vi "Limelight Aim & Range.vi"() -> (2 "Right command":dbl, 3 "left command":dbl)   [LabVIEW 2019]
uses:
  Framework/Robot Global Data.vi
panel:
  out "tv - valid target":dbl=1.0
  out "ty - offsetAngle V":dbl=-1.5031967163085938
  out "tx - offsetAngle H":dbl=0.16126251220703125
  out "distance adjust":dbl
  out "steering adjust":dbl
  out "heading error":dbl
  out "distance error":dbl
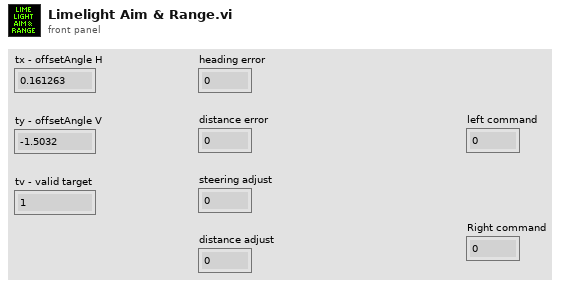
[diagram p1: front panel]
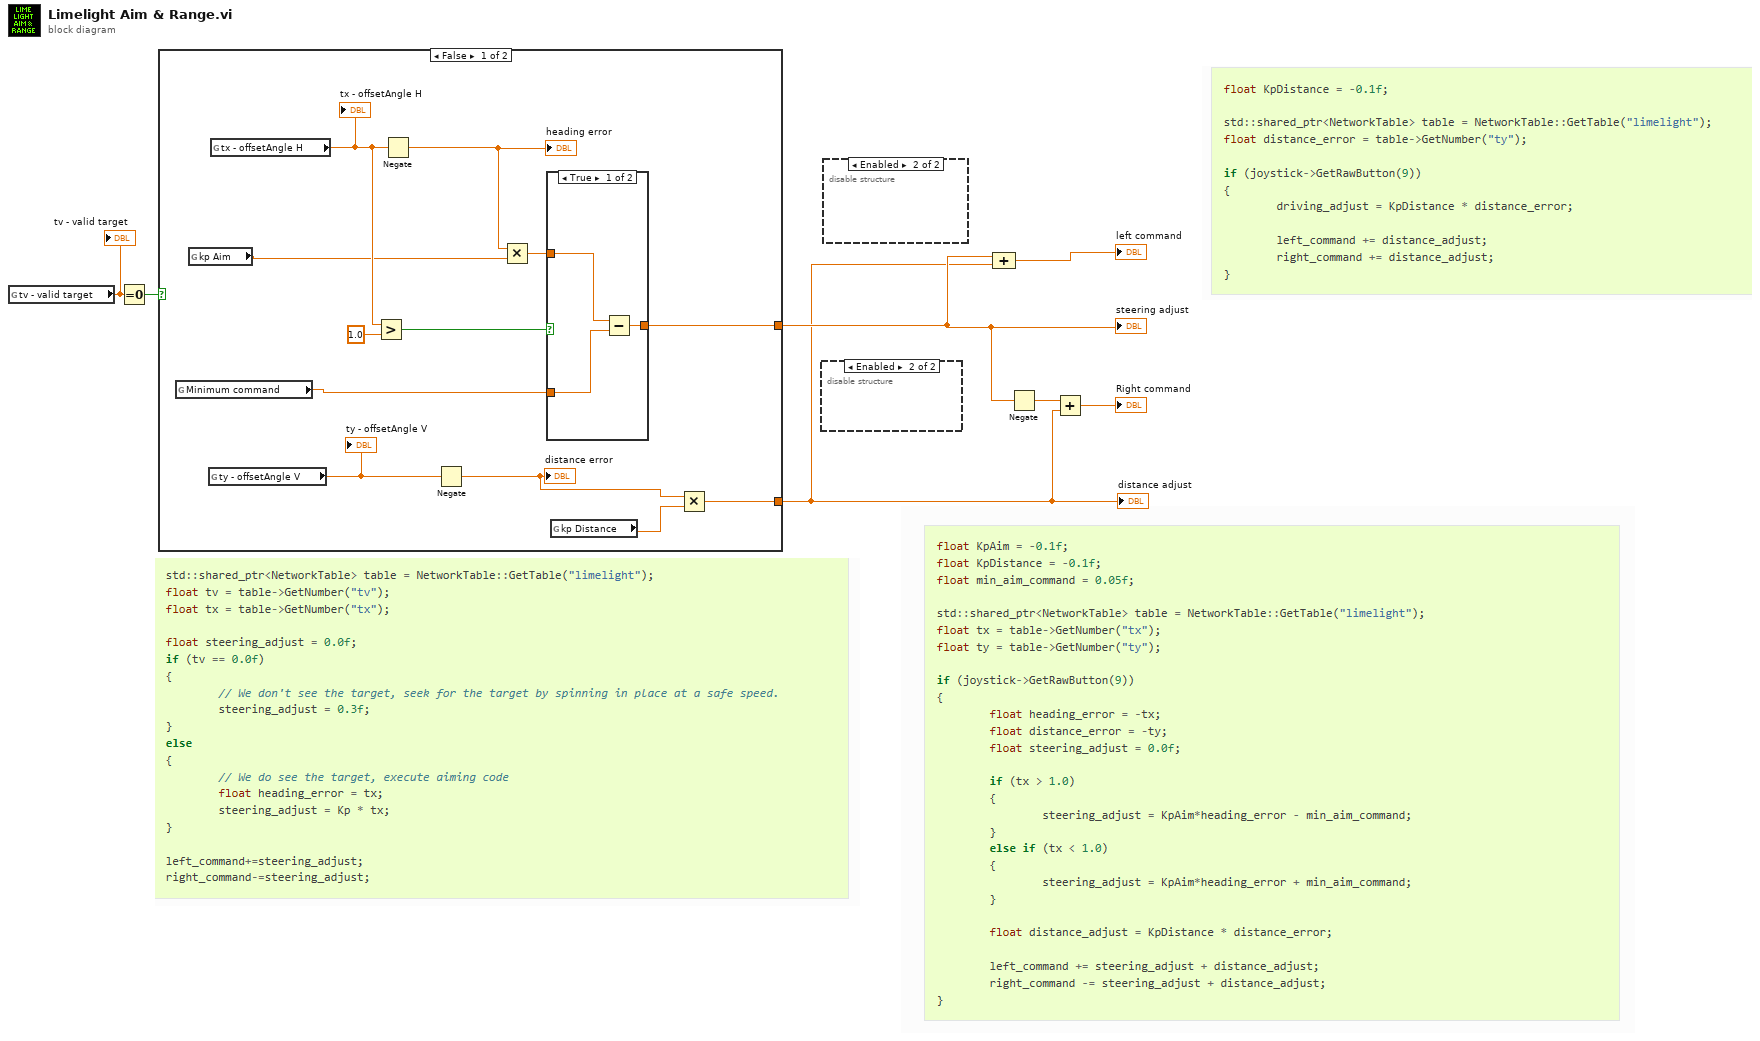
[diagram p0: block diagram]
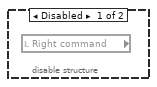
[diagram p2: hidden frame]
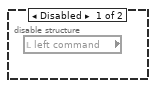
[diagram p3: hidden frame]
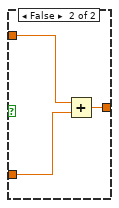
[diagram p4: hidden frame]
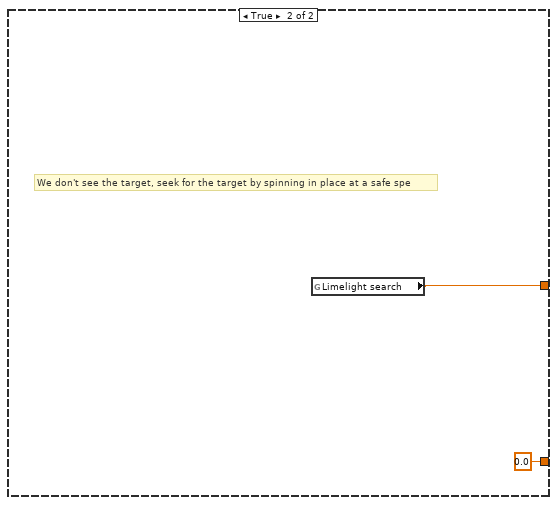
[diagram p5: hidden frame]
diagram:
  n1 = global read "Robot Global Data.vi" "tv - valid target"() -> (w1:dbl)
  "tv - valid target" <- w1
  n2 = Equal To 0?(x=w1) -> (x = 0?=w7:bool)
  n3 = case shown="False" w7 {
    tunnel: [w15 w26] -> w5
    tunnel: [w13 0.0] -> w4
    frame False {
      n4 = global read "Robot Global Data.vi" "Minimum command"() -> (w9:dbl)
      n5 = global read "Robot Global Data.vi" "kp Aim"() -> (w10:dbl)
      n6 = global read "Robot Global Data.vi" "ty - offsetAngle V"() -> (w12:dbl)
      "ty - offsetAngle V" <- w12
      n7 = global read "Robot Global Data.vi" "tx - offsetAngle H"() -> (w11:dbl)
      "tx - offsetAngle H" <- w11
      n8 = Greater?(x=w11, y=1.0) -> (0:w19:bool)
      n9 = Negate(x=w11) -> (-x=w17:dbl)
      "heading error" <- w17
      n10 = Negate(x=w12) -> (-x=w14:dbl)
      "distance error" <- w14
      n11 = Multiply(x=w17, y=w10) -> (x*y=w16:dbl)
      n12 = case shown="True" w19 {
        tunnel: w16 -> [w22 w25]
        tunnel: w9 -> [w21 w24]
        tunnel: [w20 w23] -> w15
        frame True {
          n13 = Subtract(x=w22, y=w21) -> (x-y=w20:dbl)
        }
        frame False {
          n14 = Add(x=w25, y=w24) -> (x+y=w23:dbl)
        }
      }
      n15 = global read "Robot Global Data.vi" "kp Distance"() -> (w8:dbl)
      n16 = Multiply(x=w14, y=w8) -> (x*y=w13:dbl)
    }
    frame True {
      # "We don't see the target, seek for the target by spinning in place at a safe spe"
      n17 = global read "Robot Global Data.vi" "Limelight search"() -> (w26:dbl)
    }
  }
  "steering adjust" <- w5
  "distance adjust" <- w4
  n18 = disable-structure shown="Enabled" {
    frame Disabled {
      n19 = local read "Right command"() -> ()  [unwired: 1 out]
    }
    frame Enabled {
    }
  }
  n20 = disable-structure shown="Enabled" {
    frame Disabled {
      n21 = local read "left command"() -> ()  [unwired: 1 out]
    }
    frame Enabled {
    }
  }
  n22 = Compound Arithmetic op=ADD(w5, w4) -> (→"left command":dbl)
  n23 = Negate(x=w5) -> (-x=w3:dbl)
  n24 = Add(x=w3, y=w4) -> (x+y=→"Right command":dbl)
